vi "replace_string.vi"(1 "file path":path, 2 "Replace With":string, 3 "Find Word":string) -> (0 "File":string)   [LabVIEW 2018]
doc: "This VI searches a text file for a given string (<B>Find Word</B>) and replaces it with another string (<B>Replace With</B>)."
panel:
  # "Select Help»Show Context Help and move the cursor over the VI icon to display help for this VI."
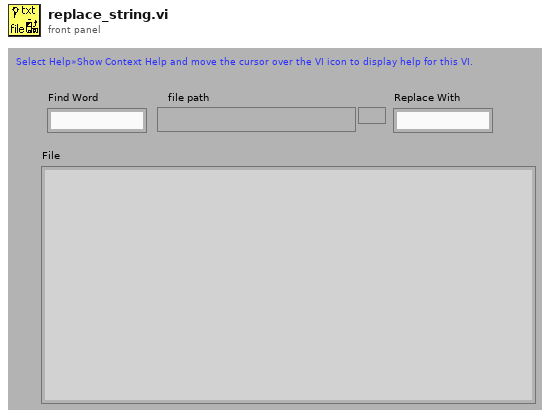
[diagram p1: front panel]
types:
  T1 = enum16{"open", "open or create", "create or replace", "create", "open (read only)"}
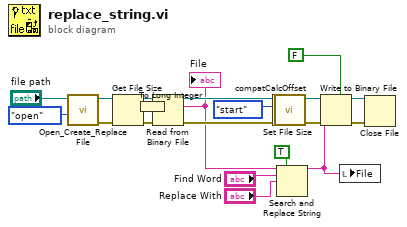
[diagram p0: block diagram]
diagram:
  n1 = call <vilib>:"Open_Create_Replace File.vi"("function (open:0)"=T1."open", "file path"="file path") -> ("error out"=w21:errorcluster, "refnum"=w22:refnum<file>)  [unwired: 6 in, 2 out]
  n2 = Get File Size(file=w22, error in=w21) -> (refnum out=w20:refnum<file>, size (in bytes)=w1:i64, 0:w19:errorcluster)
  n3 = To Long Integer(number=w1) -> (32bit integer=w18:i32)
  n4 = Read from Binary File(8:w19, 10:w18, 11:w20) -> (0:w12:errorcluster, 2:w6:string, 3:w7:refnum<file>)  [unwired: 3 in, 1 out]
  "File" <- w6
  n5 = call <vilib>:"compatCalcOffset.vi"("error in"=w12, "pos mode (0:1)"=enum16{"start", "end", "current"}."start", "refnum"=w7) -> ("error out"=w5:errorcluster, "offset"=w4:i32, "dup refnum"=w3:refnum<file>)  [unwired: 6 in]
  n6 = Set File Size(4:w5, 6:w4, 7:w3) -> (0:w13:errorcluster, 3:w14:refnum<file>)
  n7 = Search and Replace String(replace all?=TRUE ("replace all? (F)"), input string=w6, search string="Find Word", replace string="Replace With") -> (result string=w8:string)  [unwired: 4 in, 3 out]
  n8 = Write to Binary File(file (use dialog)=w14, data=w8, error in=w13, 5:FALSE ("prepend array or string size? (T)")) -> (refnum out=w15:refnum<file>, error out=w16:errorcluster)  [unwired: 2 in, 1 out]
  n9 = local write "File"(w8) -> ()
  n10 = Close File(refnum=w15, error in=w16) -> ()  [unwired: 2 out]
